vi "Write File middle.vi"(8 "error in (no error)":errorcluster, 10 "File middle":string, 11 "Worker Actor in":refnum<class "Worker Actor.lvclass">) -> (0 "error out":errorcluster, 3 "Worker Actor out":refnum<class "Worker Actor.lvclass">)   [LabVIEW 2024, in "Worker Actor.lvclass"]
uses:
  Worker Actor.lvclass
  Worker Actor.lvclass/Worker Actor.ctl
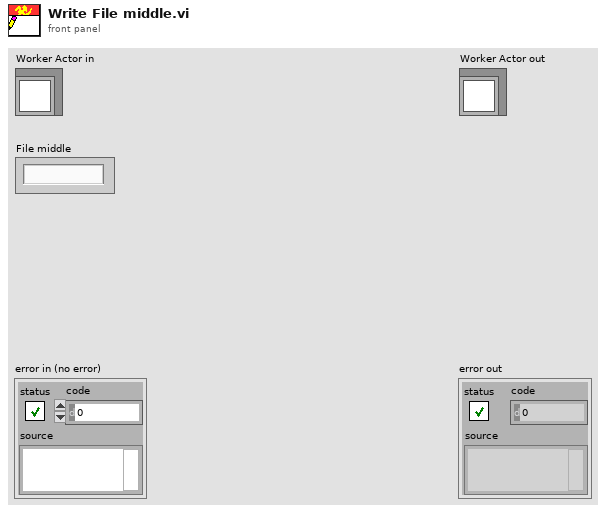
[diagram p1: front panel]
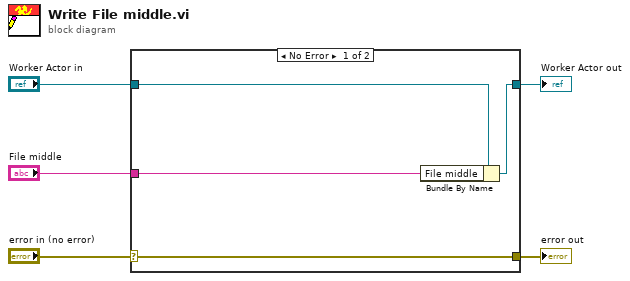
[diagram p0: block diagram]
diagram:
  n1 = case shown="No Error" "error in (no error)" {
    selector: "error in (no error)" -> [w9 w10]
    tunnel: [w9 w10] -> w4
    tunnel: [w7 w11] -> w2
    tunnel: "Worker Actor in" -> [w8 w11]
    tunnel: "File middle" -> [w6 _]
    frame No Error {
      n2 = Bundle By Name(cluster=w8, "File middle"=w6) -> (w7:refnum<class "Worker Actor.lvclass">)
    }
    frame Error {
    }
  }
  "error out" <- w4
  "Worker Actor out" <- w2
